vi "Margins.vi"(8 "error in (no error)":errorcluster, 10 "Page setup IN":T1={"Page Size"=1, "Orientation"=enum."Portrait", "Custom Size"={"Width"=0.0, "Height"=0.0}, "Margins"={"Left"=25.0, "Right"=25.0, "Top"=25.0, "Bottom"=25.0}} {"Page Size" items=["Custom", "LETTER", "NOTE", "LEGAL", "TABLOID", "EXECUTIVE", "POSTCARD", "A0", "A1", "A2", "A3", "A4", "A5", "A6", "A7", "A8", "A9", "A10", "B0", "B1", "B2", "B3", "B4", "B5", "B6", "B7", "B8", "B9", "B10", "ARCH_E", "ARCH_D", "ARCH_C", "ARCH_B", "ARCH_A", "FLSA", "FLSE", "HALFLETTER", "_11X17", "ID_1", "ID_2", "ID_3", "LEDGER", "CROWN_QUARTO", "LARGE_CROWN_QUARTO", "DEMY_QUARTO", "ROYAL_QUARTO", "CROWN_OCTAVO", "LARGE_CROWN_OCTAVO", "DEMY_OCTAVO", "ROYAL_OCTAVO", "SMALL_PAPERBACK", "PENGUIN_SMALL_PAPERBACK", "PENGUIN_LARGE_PAPERBACK"]}, 11 "Unit (default = mm)":T6=enum."mm") -> (0 "error out":errorcluster, 2 "Page setup OUT":T1={"Page Size"=1, "Orientation"=enum."Portrait", "Custom Size"={"Width"=0.0, "Height"=0.0}, "Margins"={"Left"=25.0, "Right"=25.0, "Top"=25.0, "Bottom"=25.0}} {"Page Size" items=["Custom", "LETTER", "NOTE", "LEGAL", "TABLOID", "EXECUTIVE", "POSTCARD", "A0", "A1", "A2", "A3", "A4", "A5", "A6", "A7", "A8", "A9", "A10", "B0", "B1", "B2", "B3", "B4", "B5", "B6", "B7", "B8", "B9", "B10", "ARCH_E", "ARCH_D", "ARCH_C", "ARCH_B", "ARCH_A", "FLSA", "FLSE", "HALFLETTER", "_11X17", "ID_1", "ID_2", "ID_3", "LEDGER", "CROWN_QUARTO", "LARGE_CROWN_QUARTO", "DEMY_QUARTO", "ROYAL_QUARTO", "CROWN_OCTAVO", "LARGE_CROWN_OCTAVO", "DEMY_OCTAVO", "ROYAL_OCTAVO", "SMALL_PAPERBACK", "PENGUIN_SMALL_PAPERBACK", "PENGUIN_LARGE_PAPERBACK"]}, 3 "Rectangle":refnum<k24>)   [LabVIEW 2019]
doc: "Version 1.0\nDeveloped by Jean-Marc Simard\nCopyright © 2010, Exaprom Inc.\nAll rights reserved.\nLicense: BSD\n\nWith iTextSharp 4.1.6 (http://itextsharp.sourceforge.net)\nunder Mozilla Public License Version 1.1\n(http://www.mozilla.org/MPL/MPL-1.1.html)"
uses:
  <userlib>/Exaprom PDF/Controls/Page Controls/Page setup.ctl
  <userlib>/Exaprom PDF/Controls/Page Controls/Page size.ctl
  <userlib>/Exaprom PDF/Controls/Page Controls/Page Orientation.ctl
  <userlib>/Exaprom PDF/Controls/Page Controls/Page Layout Custom.ctl
  <userlib>/Exaprom PDF/Controls/Page Controls/Page margins.ctl
  <userlib>/Exaprom PDF/Controls/Initialization Controls/Unit.ctl
  C:/Program Files/National Instruments/LabVIEW 2019/user.lib/Exaprom PDF/DLL/itextsharp.dll
  DLL/itextsharp.dll
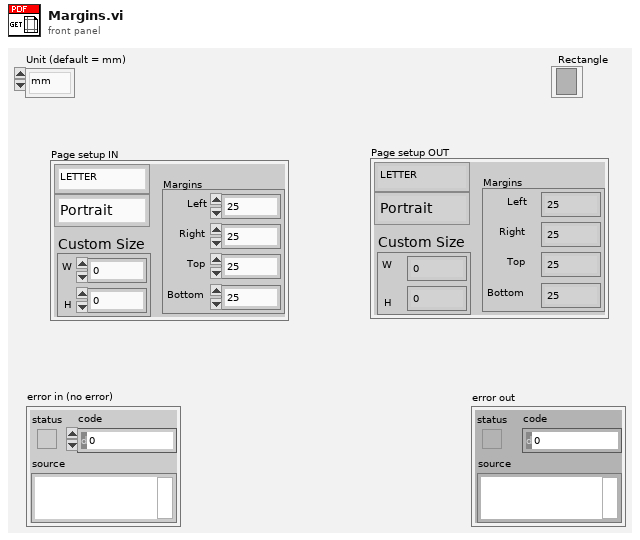
[diagram p1: front panel]
types:
  T1 = typedef "Page setup.ctl" = cluster{"Page Size":T2, "Orientation":T3, "Custom Size":T4, "Margins":T5}
  T2 = typedef "Page size.ctl" = i32
  T3 = typedef "Page Orientation.ctl" = enum16{"Portrait", "Landscape"}
  T4 = typedef "Page Layout Custom.ctl" = cluster{"Width":sgl, "Height":sgl}
  T5 = typedef "Page margins.ctl" = cluster{"Left":sgl, "Right":sgl, "Top":sgl, "Bottom":sgl}
  T6 = typedef "Unit.ctl" = enum16{"inch", "mm"}
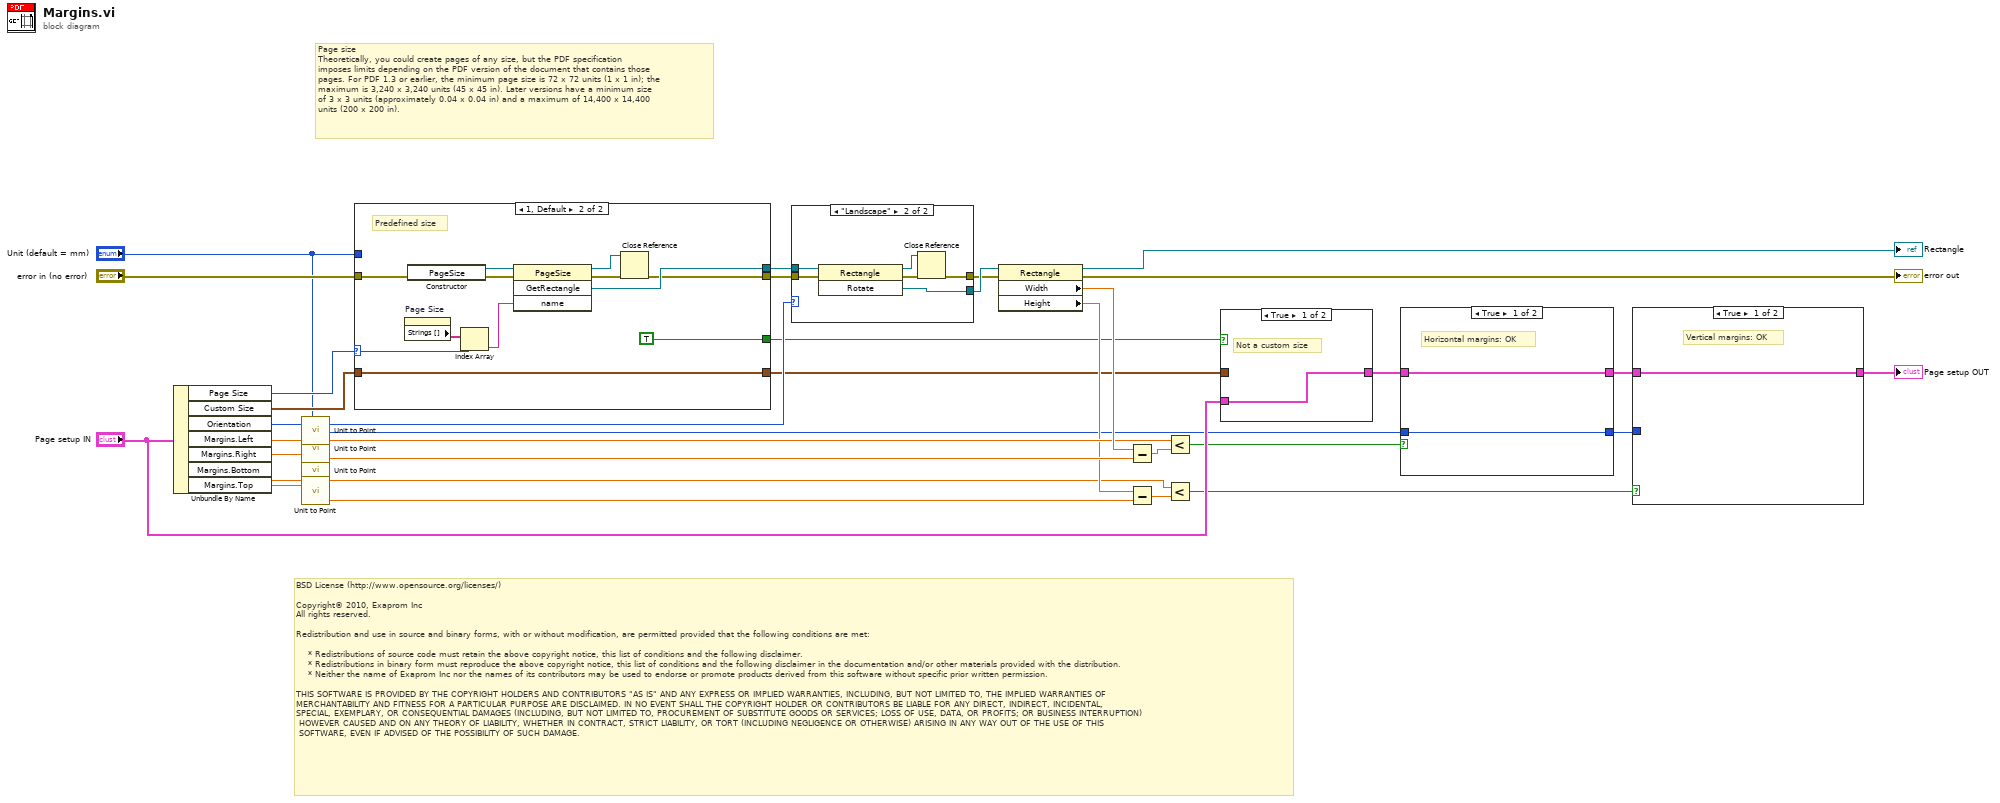
[diagram p0: block diagram]
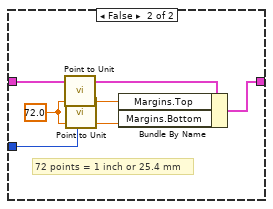
[diagram p2: hidden frame]
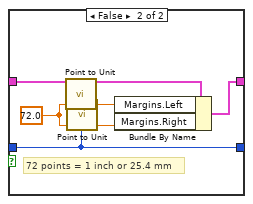
[diagram p3: hidden frame]
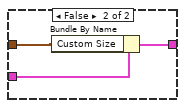
[diagram p4: hidden frame]
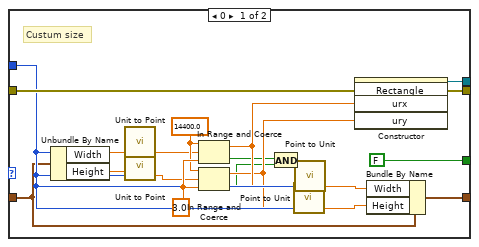
[diagram p6: hidden frame]
diagram:
  # "BSD License (http://www.opensource.org/licenses/)\n\nCopyright© 2010, Exaprom Inc\nAll rights reserved.\n\nRedistribution and use in source and binary forms, with or without modification, are permitted provided that the following conditions are met:\n\n    * Redistributions of source code must retain the above copyright notice, this list of conditions and the following disclaimer.\n    * Redistributions in binary form must reproduce the above copyright notice, this list of conditions and the following disclaimer in the documentation and/or other materials provided with the distribution.\n    * Neither the name of Exaprom Inc nor the names of its contributors may be used to endorse or promote products derived from this software without specific prior written permission.\n\nTHIS SOFTWARE IS PROVIDED BY THE COPYRIGHT HOLDERS AND CONTRIBUTORS \"AS IS\" AND ANY EXPRESS OR IMPLIED WARRANTIES, INCLUDING, BUT NOT LIMITED TO, THE IMPLIED WARRANTIES OF \nMERCHANTABILITY AND FITNESS FOR A PARTICULAR PURPOSE ARE DISCLAIMED. IN NO EVENT SHALL THE COPYRIGHT HOLDER OR CONTRIBUTORS BE LIABLE FOR ANY DIRECT, INDIRECT, INCIDENTAL,\nSPECIAL, EXEMPLARY, OR CONSEQUENTIAL DAMAGES (INCLUDING, BUT NOT LIMITED TO, PROCUREMENT OF SUBSTITUTE GOODS OR SERVICES; LOSS OF USE, DATA, OR PROFITS; OR BUSINESS INTERRUPTION)\n HOWEVER CAUSED AND ON ANY THEORY OF LIABILITY, WHETHER IN CONTRACT, STRICT LIABILITY, OR TORT (INCLUDING NEGLIGENCE OR OTHERWISE) ARISING IN ANY WAY OUT OF THE USE OF THIS\n SOFTWARE, EVEN IF ADVISED OF THE POSSIBILITY OF SUCH DAMAGE."
  # "Page size\nTheoretically, you could create pages of any size, but the PDF specification\nimposes limits depending on the PDF version of the document that contains those\npages. For PDF 1.3 or earlier, the minimum page size is 72 x 72 units (1 x 1 in); the\nmaximum is 3,240 x 3,240 units (45 x 45 in). Later versions have a minimum size\nof 3 x 3 units (approximately 0.04 x 0.04 in) and a maximum of 14,400 x 14,400\nunits (200 x 200 in)."
  n1 = Unbundle By Name("Page setup IN") -> ("Page Size"=w32:T2, "Custom Size"=w31:T4, "Orientation"=w25:T3, "Margins.Left"=w29:sgl, "Margins.Right"=w28:sgl, "Margins.Bottom"=w27:sgl, "Margins.Top"=w26:sgl)
  n2 = call <userlib>:"Unit to Point.vi"("X unit"=w29, "Unit (default = mm)"="Unit (default = mm)") -> ("X point"=w18:sgl)  [unwired: 7 out]
  n3 = call <userlib>:"Unit to Point.vi"("X unit"=w28, "Unit (default = mm)"="Unit (default = mm)") -> ("X point"=w19:sgl)  [unwired: 7 out]
  n4 = call <userlib>:"Unit to Point.vi"("X unit"=w27, "Unit (default = mm)"="Unit (default = mm)") -> ("X point"=w15:sgl)  [unwired: 7 out]
  n5 = call <userlib>:"Unit to Point.vi"("X unit"=w26, "Unit (default = mm)"="Unit (default = mm)") -> ("X point"=w14:sgl)  [unwired: 7 out]
  n6 = case shown="1, Default" w32 {
    selector: w32 -> [_ w60]
    tunnel: [w51 w55] -> w30
    tunnel: [w50 w63] -> w2
    tunnel: w31 -> [w36 w53]
    tunnel: "error in (no error)" -> [w49 w54]
    tunnel: "Unit (default = mm)" -> [w42 _]
    tunnel: [w37 w53] -> w12
    tunnel: [FALSE TRUE] -> w11
    frame 0 {
      w47 = sgl 14400.0
      w48 = sgl 3.0
      # "Custum size"
      n7 = Unbundle By Name(w36) -> ("Width"=w46:sgl, "Height"=w45:sgl)
      n8 = call <userlib>:"Unit to Point.vi"("X unit"=w46, "Unit (default = mm)"=w42) -> ("X point"=w43:sgl)  [unwired: 7 out]
      n9 = call <userlib>:"Unit to Point.vi"("X unit"=w45, "Unit (default = mm)"=w42) -> ("X point"=w44:sgl)  [unwired: 7 out]
      n10 = In Range and Coerce(upper limit=w47, x=w43, lower limit=w48) -> (coerced(x)=w41:sgl, In Range?=w35:bool)
      n11 = In Range and Coerce(upper limit=w47, x=w44, lower limit=w48) -> (coerced(x)=w40:sgl, In Range?=w34:bool)
      n12 = And(x=w35, y=w34) -> ()  [unwired: 1 out]
      n13 = call <userlib>:"Point to Unit.vi"("X point"=w40, "Unit (default = mm)"=w42) -> ("X unit"=w38:sgl)  [unwired: 7 out]
      n14 = call <userlib>:"Point to Unit.vi"("X point"=w41, "Unit (default = mm)"=w42) -> ("X unit"=w39:sgl)  [unwired: 7 out]
      n15 = constructor class="Rectangle"(error in=w49, "urx"=w41, "ury"=w40) -> (reference out=w50:refnum<k24>, error out=w51:errorcluster)  [unwired: 2 in, 3 out]
      n16 = Bundle By Name(cluster=w36, "Width"=w39, "Height"=w38) -> (w37:T4)
    }
    frame 1, Default {
      # "Predefined size"
      n17 = property on="Page Size" class="Ring (strict)"() -> ("Strings []"=w61:string[])  [unwired: 2 in, 2 out]
      n18 = constructor class="PageSize"(error in=w54) -> (reference out=w59:refnum<k24>, error out=w58:errorcluster)  [unwired: 2 in, 1 out]
      n19 = Index Array(array=w61, index=w60) -> (element=w62:string)
      n20 = invoke class="PageSize" method="GetRectangle"(reference=w59, error in=w58, "name"=w62) -> (reference out=w56:refnum<k24>, error out=w57:errorcluster, "GetRectangle"=w63:refnum<k24>)  [unwired: 1 in, 1 out]
      n21 = Close Reference(reference=w56, error in (no error)=w57) -> (error out=w55:errorcluster)
    }
  }
  n22 = case shown="\"Landscape\"" w25 {
    tunnel: [w64 w66] -> w21
    tunnel: [w65 w71] -> w24
    tunnel: w2 -> [w65 w70]
    tunnel: w30 -> [w64 w69]
    frame "Portrait", Default {
    }
    frame "Landscape" {
      n23 = invoke class="Rectangle" method="Rotate"(reference=w70, error in=w69) -> (reference out=w67:refnum<k24>, error out=w68:errorcluster, "Rotate"=w71:refnum<k24>)  [unwired: 1 in]
      n24 = Close Reference(reference=w67, error in (no error)=w68) -> (error out=w66:errorcluster)
    }
  }
  n25 = property class="Rectangle"(reference=w24, error in=w21) -> (reference out=→"Rectangle":refnum<k24>, error out=→"error out":errorcluster, "Width"=w20:sgl, "Height"=w16:sgl)
  n26 = Subtract(x=w20, y=w19) -> (x-y=w17:sgl)
  n27 = Subtract(x=w16, y=w14) -> (x-y=w13:sgl)
  n28 = Less?(x=w18, y=w17) -> (x < y?=w9:bool)
  n29 = Less?(x=w15, y=w13) -> (x < y?=w4:bool)
  n30 = case shown="True" w11 {
    tunnel: [w72 w75] -> w8
    tunnel: w12 -> [_ w74]
    tunnel: "Page setup IN" -> [w72 w73]
    frame True {
      # "Not a custom size"
    }
    frame False {
      n31 = Bundle By Name(cluster=w73, "Custom Size"=w74) -> (w75:T1)
    }
  }
  n32 = case shown="True" w9 {
    tunnel: [w77 w80] -> w6
    tunnel: w8 -> [w77 w79]
    tunnel: "Unit (default = mm)" -> [w76 w78]
    tunnel: [w76 w78] -> w7
    frame True {
      # "Horizontal margins: OK"
    }
    frame False {
      w83 = sgl 72.0 ("X point")
      # "72 points = 1 inch or 25.4 mm"
      n33 = call <userlib>:"Point to Unit.vi"("X point"=w83, "Unit (default = mm)"=w78) -> ("X unit"=w81:sgl)  [unwired: 7 out]
      n34 = call <userlib>:"Point to Unit.vi"("X point"=w83, "Unit (default = mm)"=w78) -> ("X unit"=w82:sgl)  [unwired: 7 out]
      n35 = Bundle By Name(cluster=w79, "Margins.Left"=w81, "Margins.Right"=w82) -> (w80:T1)
    }
  }
  n36 = case shown="True" w4 {
    tunnel: [w84 w87] -> w5
    tunnel: w6 -> [w84 w86]
    tunnel: w7 -> [_ w85]
    frame True {
      # "Vertical margins: OK"
    }
    frame False {
      w90 = sgl 72.0 ("X point")
      # "72 points = 1 inch or 25.4 mm"
      n37 = call <userlib>:"Point to Unit.vi"("X point"=w90, "Unit (default = mm)"=w85) -> ("X unit"=w88:sgl)  [unwired: 7 out]
      n38 = call <userlib>:"Point to Unit.vi"("X point"=w90, "Unit (default = mm)"=w85) -> ("X unit"=w89:sgl)  [unwired: 7 out]
      n39 = Bundle By Name(cluster=w86, "Margins.Top"=w88, "Margins.Bottom"=w89) -> (w87:T1)
    }
  }
  "Page setup OUT" <- w5
